vi "serial.vi"(0 "VISA resource name":refnum<visa-resource-name>="COM3", 5 "baud rate":u32=230400, 9 "delay before read (ms)":u32=500) -> ()   [LabVIEW 2015]
doc: "The Basic Serial Read and Write example performs a Serial Port Read, a Serial Port Write, or a combination of these actions. The user selects the actions (read or write) on the front panel. If both are selected, the VI will write the data first, read data, and then close the VISA session that is opened to the port. This VI will wait until the specified number of bytes is received at the port or until a termination character is read.\n\nINSTRUCTIONS:\n1) Select the serial resource and configuration parameters (baud rate, data bits, parity, stop bits, flow control).\n2) Select the operations to be performed. \n3) Connect the serial port to your device. If no device is available, perform a loopback test by doing one of the following. Short pins 2 and 3 on a RS-232 cable or short pin 4 to pin 8 and pin 5 to pin 9 on a RS-485/422 cable. \n4) Run the VI to see the data read. (The \"read string\" will match the \"string to write\" if a loopback test was performed.)\n\nNote: The parameters set for the serial port must match the parameters of the connected instrument or device. In this example, the bytes to read parameter specifies the number of bytes that the serial port reads. If there were more bytes at the port than the number specified in bytes to read, those bytes would not be read. Also, if you specify to read more bytes than the number of bytes actually read, you might receive a timeout error message.\n\nOn the block diagram, the Configure Serial Port VI sets the configuration parameters. The front panel displays the controls used to configure the basic parameters, such as baud rate, data bits, and parity. Constants configure the other parameters the user probably does not need set. After the VISA Configure Serial Port VI opens the VISA session and configures the port, the VI passes the VISA resource name to other VIs that perform operations on that VISA resource. The VISA Write function sends a command to the serial device and the VISA Read function returns data based on the command. The VISA Close function then closes the reference to the serial device. It is important to close the reference; otherwise communication through with that port through protocols other than VISA might not be possible."
uses:
  <vilib>/Instr/_visa.llb/VISA Configure Serial Port (Instr).vi
panel:
  in  "Time Stamp":timestamp
  in  "Test waveform":string(combo)="1"
  out "errorout":errorcluster
  in  "Current Frequency":dbl min=0.0 step=1.0 format="%#.8g"
  in  "stop 2":bool
  in  "termination char\n(0xA = '\\n' = LF)":u8=13 format="%.0x"
  in  "flow control":u16(ring) items=["None"=0, "XON/XOFF"=1, "RTS/CTS"=2, "DTR/DSR"=4]
  in  "stop bits":u16(ring)=10 items=["1.0"=10, "1.5"=15, "2.0"=20]
  in  "parity":u16(ring) items=["None", "Odd", "Even", "Mark", "Space"]
  in  "data bits":u16=8 min=5 max=8 step=1
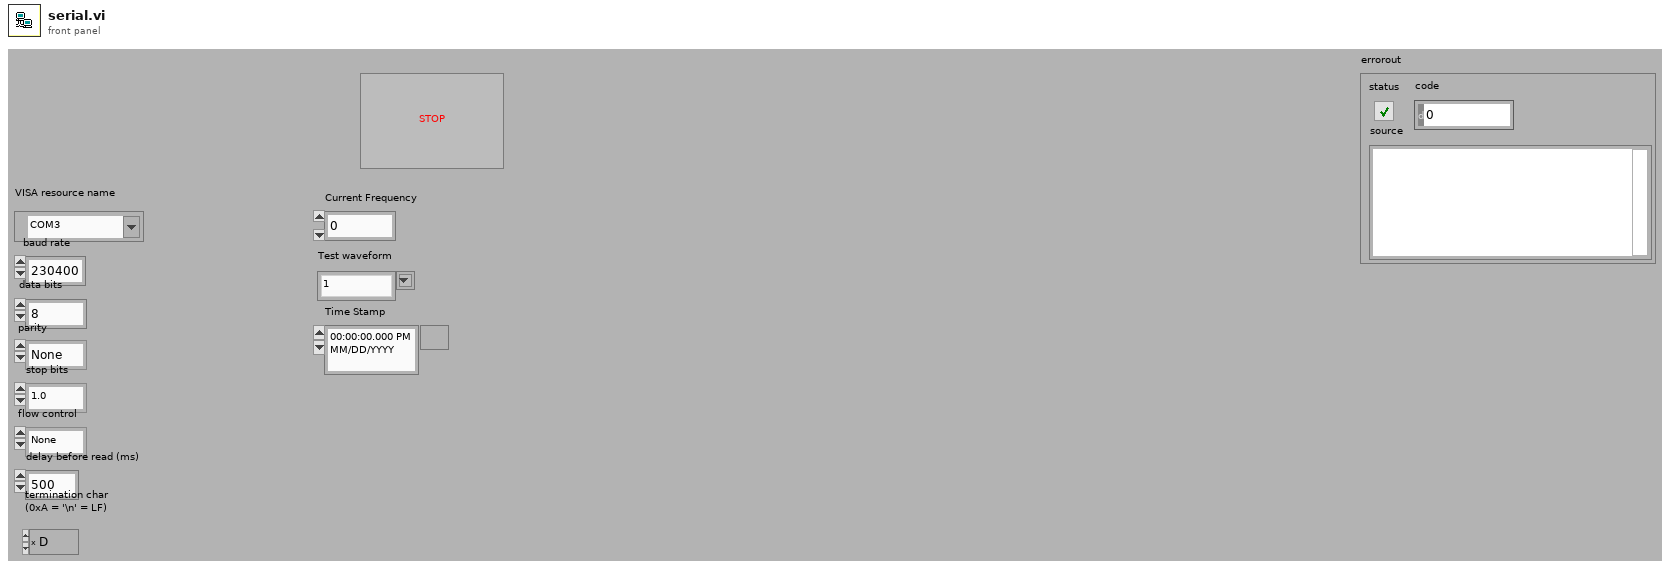
[diagram p1: front panel]
types:
  T1 = cluster{"second":i32, "minute":i32, "hour":i32, "day of month":i32, "month":i32, "year":i32, "day of week":i32, "day of year":i32, "is DST":i32}
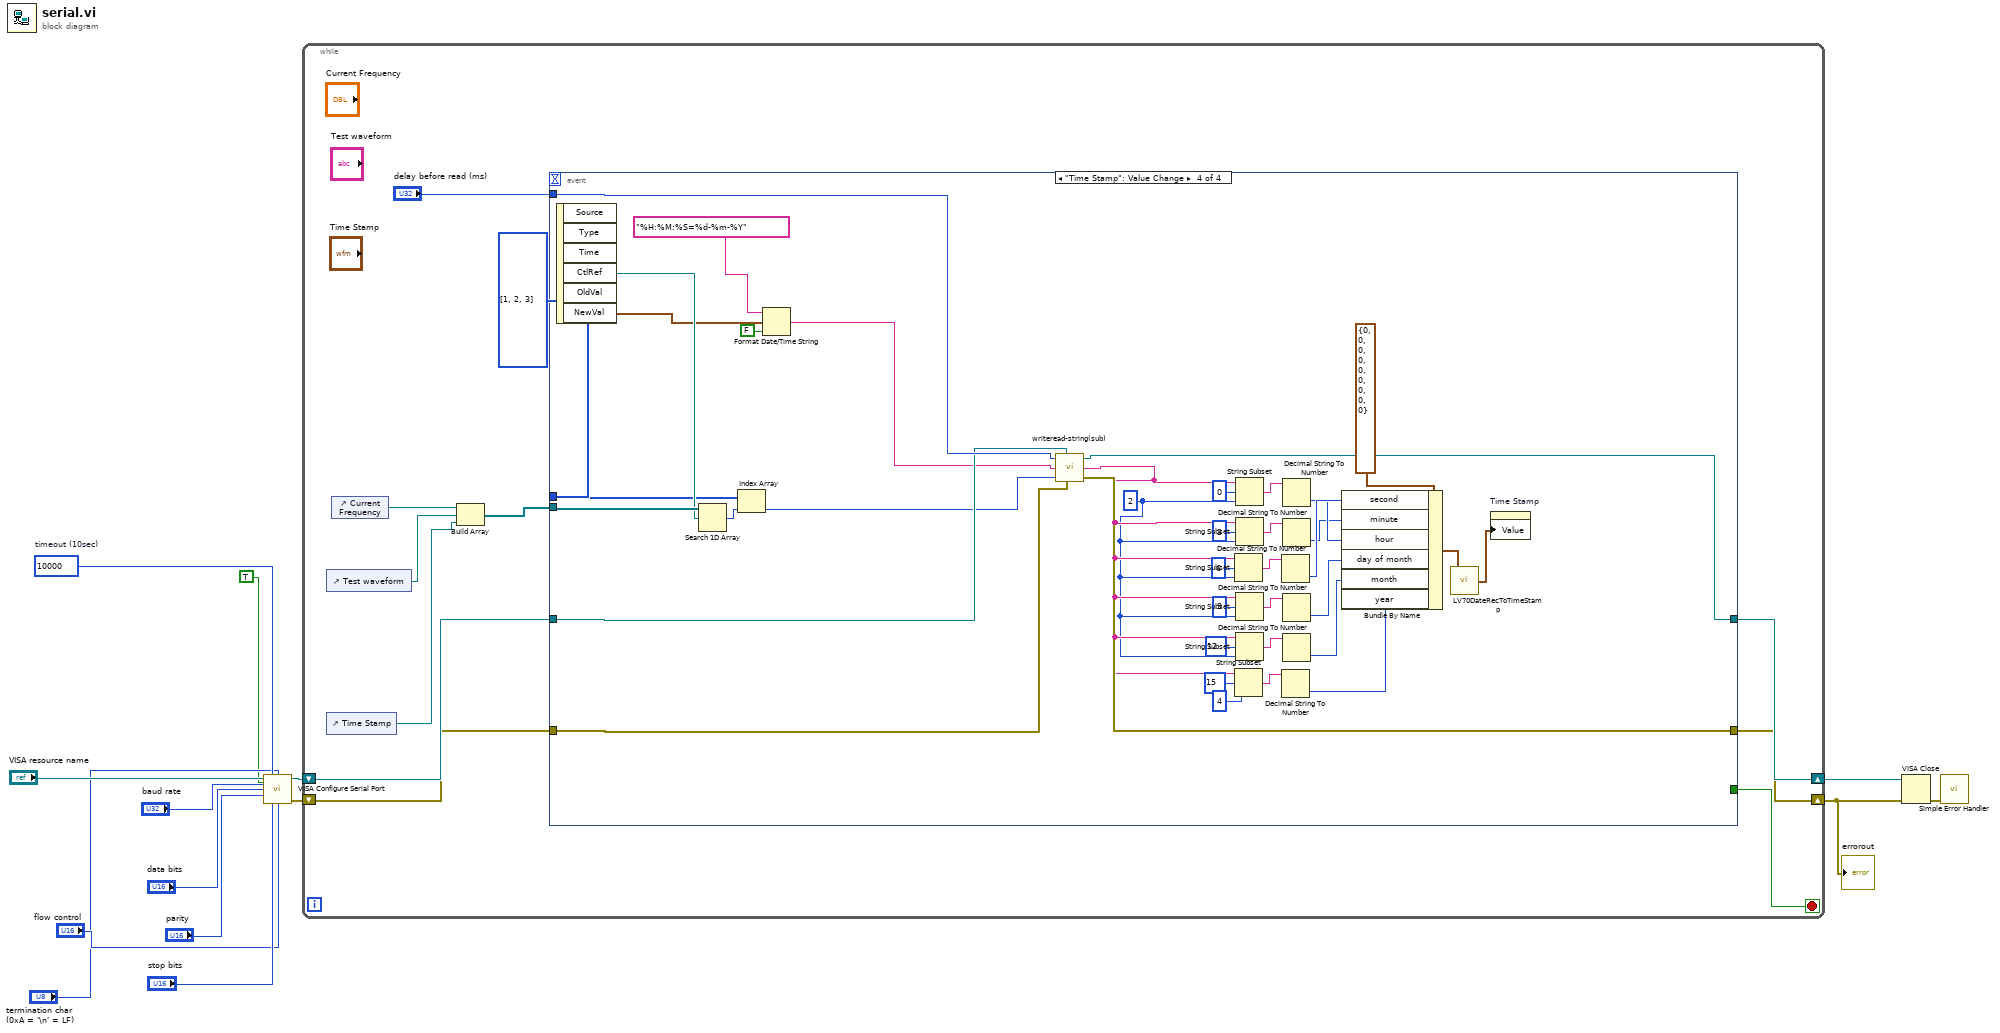
[diagram p0: block diagram]
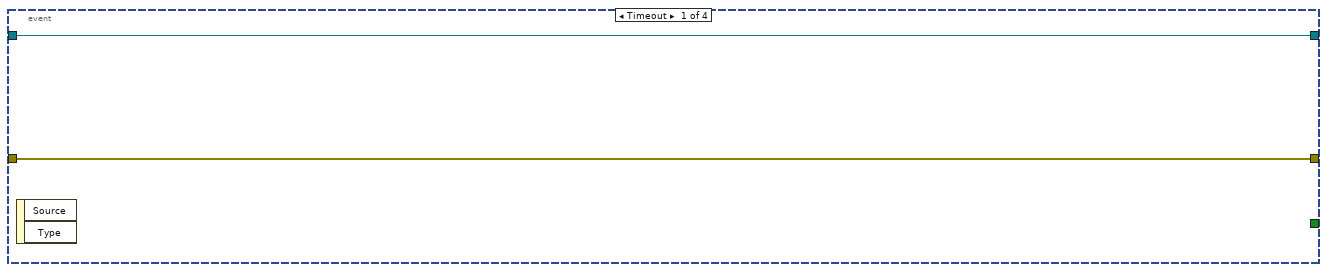
[diagram p2: hidden frame]
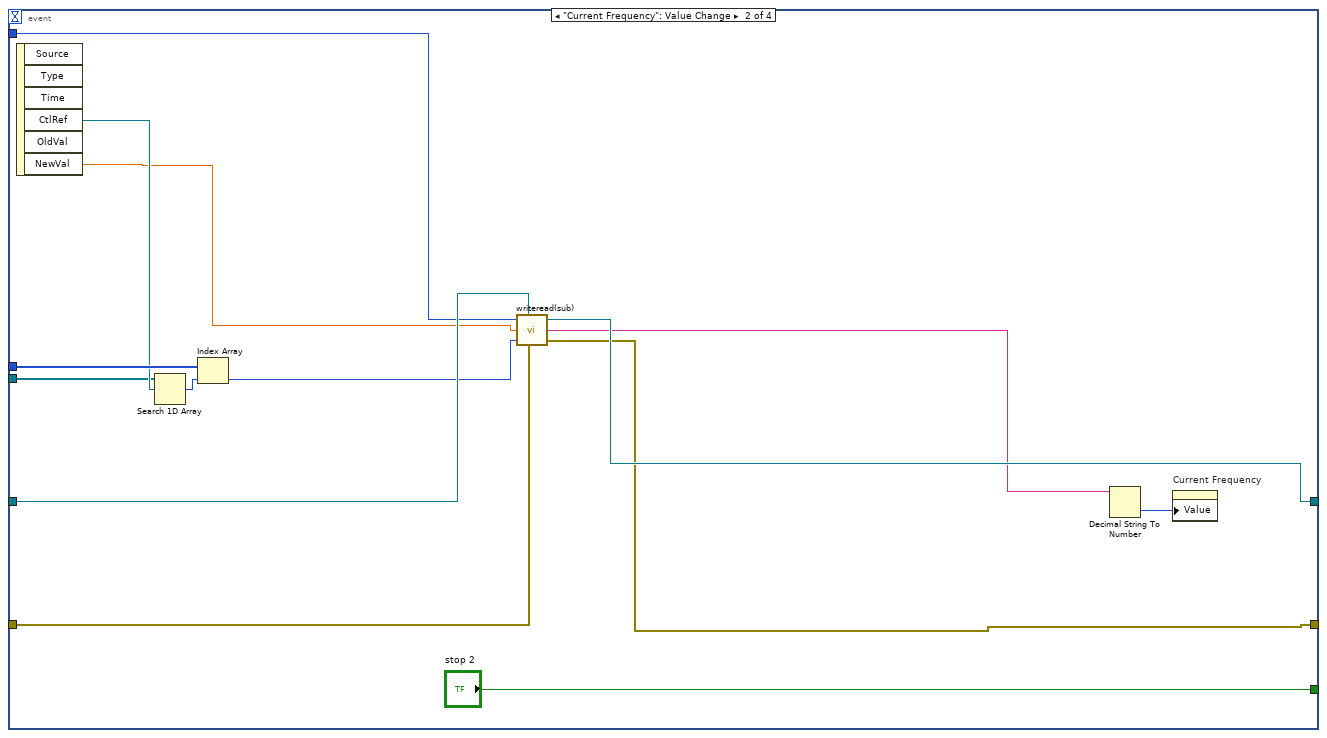
[diagram p3: hidden frame]
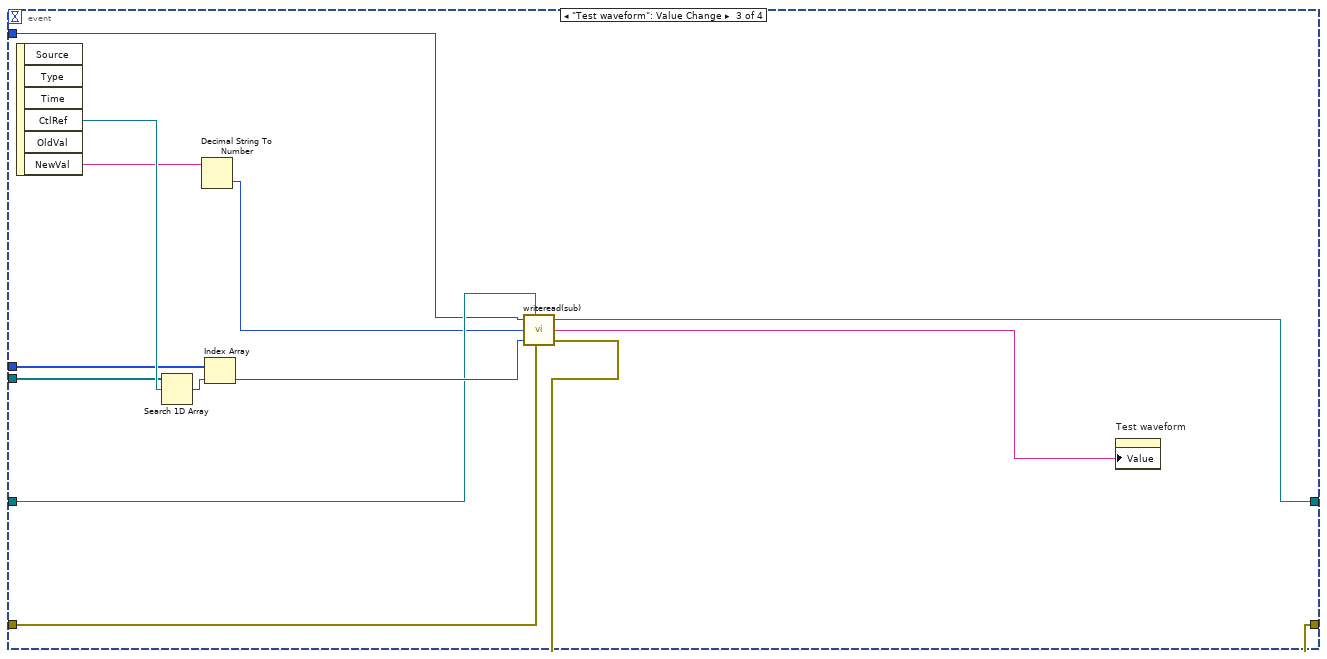
[diagram p4: hidden frame]
diagram:
  w10 = u32 10000  # timeout (10sec)
  n1 = call-poly "VISA Configure Serial Port"("VISA resource name"="VISA resource name", "timeout (10sec)"=w10, "termination char\n(0xA = '\\n' = LF)"="termination char\n(0xA = '\\n' = LF)", "Enable Termination\nChar (T)"=TRUE ("Enable Termination\nChar (T)"), "baud rate (9600)"="baud rate", "data bits (8)"="data bits", "parity (0:none)"="parity", "stop bits (10: 1 bit)"="stop bits", "flow control (0:none)"="flow control") -> ("VISA resource name out"=w3:refnum<visa-resource-name>, "error out"=w2:errorcluster)  [unwired: 1 in, 4 out]
  n2 = while {
    shift-right: [w20] -> w4
    shift-left: w3 -> [w22]
    shift-right: [w19] -> w1
    shift-left: w2 -> [w21]
    stop <- w18 stop-if-true
    n3 = control-ref of="Test waveform"() -> (w17:refnum<vi>)
    n4 = control-ref of="Time Stamp"() -> (w15:refnum<vi>)
    n5 = control-ref of="Current Frequency"() -> (w25:refnum<vi>)
    n6 = Build Array(w25, w17, w15) -> (w24:refnum<vi>[])
    n7 = event shown="[3] \"Time Stamp\": Value Change" {
      selector: _ -> [_ _ _ _]
      dyn-events: _ -> [_ _ _ _]
      timeout: _ -> [_ _ _ _]
      tunnel: w24 -> [_ w39 w50 w91]
      tunnel: i32[] [1, 2, 3] -> [_ w41 w49 w89]
      tunnel: w22 -> [w26 w35 w52 w84]
      tunnel: w21 -> [w27 w34 w48 w81]
      tunnel: [w26 w31 w45 w79] -> w20
      tunnel: [w27 w30 w46 w80] -> w19
      tunnel: [_ "stop 2" _ _] -> w18
      tunnel: "delay before read (ms)" -> [_ w28 w47 w85]
      event Timeout {
        n8 = event-data() -> ()  [unwired: 1 in, 2 out]
      }
      event "Current Frequency": Value Change {
        n9 = event-data() -> ("CtlRef"=w40:refnum<vi>, "NewVal"=w32:dbl)  [unwired: 1 in, 4 out]
        n10 = Search 1D Array(1D array=w39, element=w40) -> (index of element=w38:i32)  [unwired: 1 in]
        n11 = Index Array(array=w41, index=w38) -> (element=w33:i32)
        n12 = call "writeread(sub).vi"("delay before read (ms)"=w28, "resourcein"=w35, "New Value"=w32, "Command"=w33, "errorin"=w34) -> ("resourceout"=w31:refnum<visa-resource-name>, "readstring"=w29:string, "errorout"=w30:errorcluster)
        n13 = Decimal String To Number(string=w29) -> (number=w37:i32)  [unwired: 2 in, 1 out]
        n14 = property on="Current Frequency" class="DigNum (strict)"("Value"=w37) -> ()  [unwired: 2 in, 2 out]
      }
      event "Test waveform": Value Change {
        n15 = event-data() -> ("CtlRef"=w51:refnum<vi>, "NewVal"=w44:string)  [unwired: 1 in, 4 out]
        n16 = Search 1D Array(1D array=w50, element=w51) -> (index of element=w54:i32)  [unwired: 1 in]
        n17 = Decimal String To Number(string=w44) -> (number=w43:i32)  [unwired: 2 in, 1 out]
        n18 = Index Array(array=w49, index=w54) -> (element=w53:i32)
        n19 = call "writeread(sub).vi"("delay before read (ms)"=w47, "resourcein"=w52, "New Value"=w43, "Command"=w53, "errorin"=w48) -> ("resourceout"=w45:refnum<visa-resource-name>, "readstring"=w42:string, "errorout"=w46:errorcluster)
        n20 = property on="Test waveform" class="CmbBox"("Value"=w42) -> ()  [unwired: 2 in, 2 out]
      }
      event "Time Stamp": Value Change {
        w64 = 2 ("length (rest)")
        n21 = event-data() -> ("CtlRef"=w90:refnum<vi>, "NewVal"=w88:timestamp)  [unwired: 1 in, 4 out]
        n22 = Search 1D Array(1D array=w91, element=w90) -> (index of element=w92:i32)  [unwired: 1 in]
        n23 = Index Array(array=w89, index=w92) -> (element=w82:i32)
        n24 = Format Date/Time String(time format string (%c)="%H:%M:%S=%d-%m-%Y", seconds (now)=w88, UTC format=FALSE) -> (date/time string=w83:string)
        n25 = call "writeread-string(sub).vi"("delay before read (ms)"=w85, "resourcein"=w84, "payload"=w83, "Command"=w82, "errorin"=w81) -> ("resourceout"=w79:refnum<visa-resource-name>, "readstring"=w65:string, "errorout"=w80:errorcluster)
        n26 = String Subset(string=w65, offset (0)=6, length (rest)=w64) -> (substring=w73:string)
        n27 = String Subset(string=w65, offset (0)=15, length (rest)=4 ("length (rest)")) -> (substring=w67:string)
        n28 = String Subset(string=w65, offset (0)=0, length (rest)=w64) -> (substring=w77:string)
        n29 = String Subset(string=w65, offset (0)=3, length (rest)=w64) -> (substring=w75:string)
        n30 = String Subset(string=w65, offset (0)=9, length (rest)=w64) -> (substring=w71:string)
        n31 = String Subset(string=w65, offset (0)=12, length (rest)=w64) -> (substring=w69:string)
        n32 = Decimal String To Number(string=w73) -> (number=w60:i32)  [unwired: 2 in, 1 out]
        n33 = Decimal String To Number(string=w67) -> (number=w55:i32)  [unwired: 2 in, 1 out]
        n34 = Decimal String To Number(string=w77) -> (number=w59:i32)  [unwired: 2 in, 1 out]
        n35 = Decimal String To Number(string=w75) -> (number=w58:i32)  [unwired: 2 in, 1 out]
        n36 = Decimal String To Number(string=w71) -> (number=w57:i32)  [unwired: 2 in, 1 out]
        n37 = Decimal String To Number(string=w69) -> (number=w56:i32)  [unwired: 2 in, 1 out]
        n38 = Bundle By Name(cluster=T1 {"second"=0, "minute"=0, "hour"=0, "day of month"=0, "month"=0, "year"=0, "day of week"=0, "day of year"=0, "is DST"=0} ("date time rec"), "second"=w60, "minute"=w58, "hour"=w59, "day of month"=w57, "month"=w56, "year"=w55) -> (w62:T1)
        n39 = call <vilib>:"LV70DateRecToTimeStamp.vi"("date time rec"=w62) -> ("Time Stamp"=w61:timestamp)
        n40 = property on="Time Stamp" class="AbsTime (strict)"("Value"=w61) -> ()  [unwired: 2 in, 2 out]
      }
    }
  }
  "errorout" <- w1
  n41 = VISA Close(VISA resource name=w4, error in (no error)=w1) -> (error out=w12:errorcluster)
  n42 = call <vilib>:"Simple Error Handler.vi"("error in (no error)"=w12) -> ()  [unwired: 1 in, 8 out]
